vi "updateTime.vi"(8 "error in (no error)":errorcluster, 10 "Actuator Active Time":dbl, 11 "Data (in)":T7) -> (0 "error out":errorcluster, 3 "Data (out)":T7)   [LabVIEW 2015]
doc: "Compute the necessary delay time based on the actuator's active cycle and add it to the current time to ensure a necessary delay is made in the future (if required)."
uses:
  <vilib>/MakerHub/LINX/Private/Type Defs/LINX Ref.ctl
  <vilib>/MakerHub/LINX/Private/Type Defs/Platform.ctl
  <vilib>/MakerHub/LINX/Private/Type Defs/Interface.ctl
  <vilib>/MakerHub/LINX/Private/Device/Type Defs/LINX Device Config.ctl
  <vilib>/MakerHub/LINX/Private/Device/Type Defs/TCP Config.ctl
  <vilib>/MakerHub/LINX/Private/Device/Type Defs/Channels.ctl
  <vilib>/MakerHub/LINX/LMH-LINX.lvlib
  <vilib>/MakerHub/LINX/Private/Device/Device.lvlib
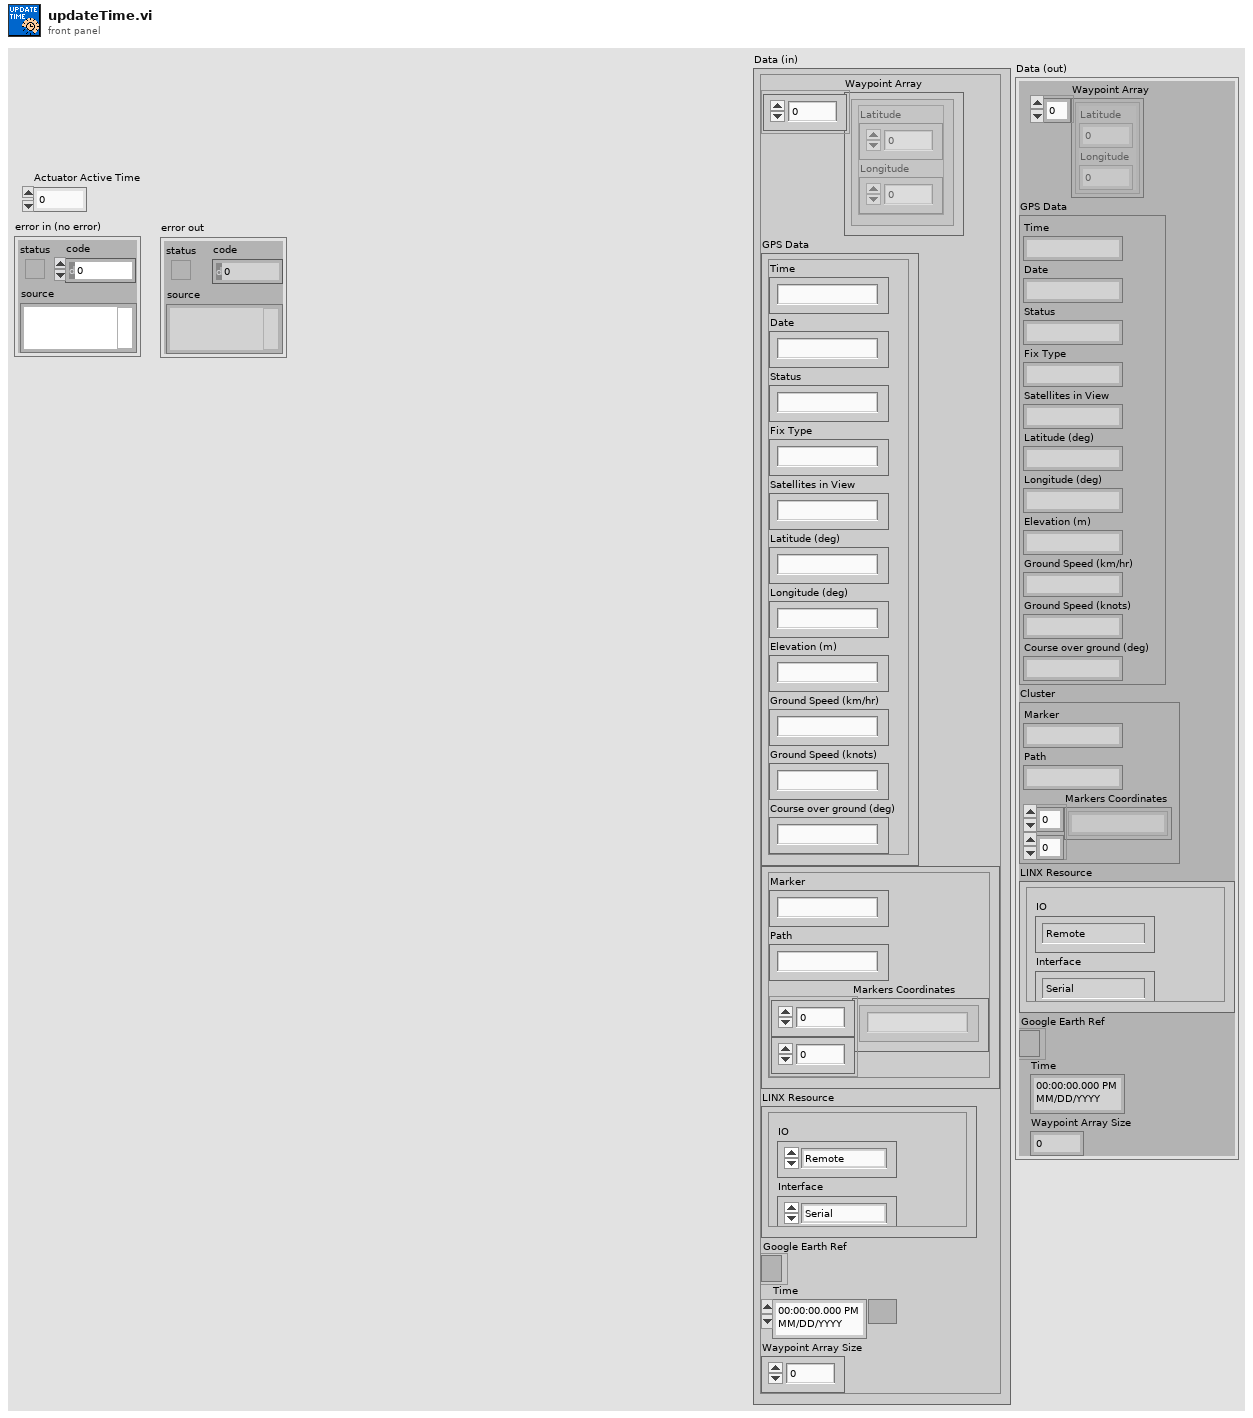
[diagram p1: front panel]
types:
  T1 = typedef "LMH-LINX.lvlib/LINX Ref.ctl" = cluster{"IO":T2, "Interface":T3, "LINX Device Config":T4}
  T2 = typedef "LMH-LINX.lvlib/Platform.ctl" = enum16{"Remote", "Local"}
  T3 = typedef "LMH-LINX.lvlib/Interface.ctl" = enum16{"Serial", "TCP"}
  T4 = typedef "LMH-LINX.lvlib/Device.lvlib/LINX Device Config.ctl" = cluster{"Interface":T3, "COM Port":refnum<visa-resource-name>, "TCP Configuration":T5, "Device Family":u8, "Device ID":u8, "Device Name":string, "TCP Ref":refnum<k5>, "Channels":T6}
  T5 = typedef "LMH-LINX.lvlib/Device.lvlib/TCP Config.ctl" = cluster{"IP Address":string, "Port":u16}
  T6 = typedef "LMH-LINX.lvlib/Channels.ctl" = cluster{"DI":u8[], "DO":u8[], "AI":u8[], "AO":u8[], "PWM":u8[], "QE":u8[], "UART":u8[], "I2C 2":u8[], "SPI":u8[], "CAN":u8[], "Servo":u8[], "AI Ref (V)":dbl, "AI Resolution (Bits)":u8, "AO Ref (V)":dbl, "AO Resolution (Bits)":u8}
  T7 = cluster{"Waypoint Array":cluster{"Latitude":dbl, "Longitude":dbl}[], "GPS Data":cluster{"Time":string, "Date":string, "Status":string, "Fix Type":string, "Satellites in View":string, "Latitude (deg)":string, "Longitude (deg)":string, "Elevation (m)":string, "Ground Speed (km/hr)":string, "Ground Speed (knots)":string, "Course over ground (deg)":string}, "Cluster":cluster{"Marker":string, "Path":string, "Markers Coordinates":string[][]}, "LINX Resource":T1, "Google Earth Ref":refnum<k7>, "Time":timestamp, "Waypoint Array Size":i32}
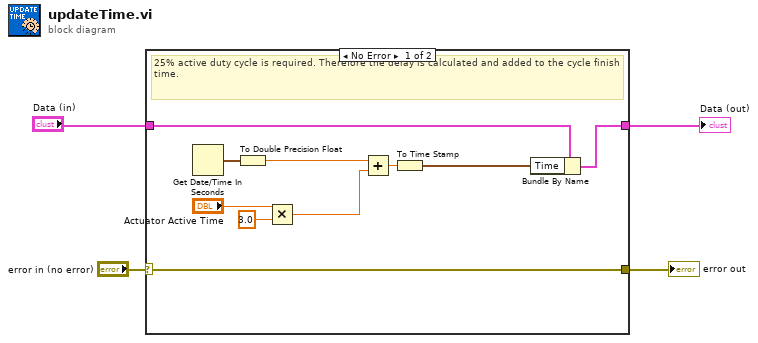
[diagram p0: block diagram]
diagram:
  n1 = case shown="No Error" "error in (no error)" {
    selector: "error in (no error)" -> [w14 w16]
    tunnel: [w14 w16] -> w4
    tunnel: "Data (in)" -> [w13 w15]
    tunnel: [w12 w15] -> w1
    frame No Error {
      # "25% active duty cycle is required. Therefore the delay is calculated and added to the cycle finish time."
      n2 = Get Date/Time In Seconds() -> (seconds since 1Jan1904=w11:timestamp)
      n3 = To Double Precision Float(number=w11) -> (double precision float=w8:dbl)
      n4 = Multiply(x="Actuator Active Time", y=3.0) -> (x*y=w7:dbl)
      n5 = Add(x=w8, y=w7) -> (x+y=w6:dbl)
      n6 = To Time Stamp(1:w6) -> (0:w5:timestamp)
      n7 = Bundle By Name(cluster=w13, "Time"=w5) -> (w12:T7)
    }
    frame Error {
    }
  }
  "error out" <- w4
  "Data (out)" <- w1
